vi "QI_correlation_X.vi"(6 "拟合半径":i32=5, 11 "QI 传递变量":T1) -> (3 "最相关位置":dbl)   [LabVIEW 2017]
doc: "本VI是QI算法中的核心部分之一，用途在于将x轴上的radial profile 连起来，并和自己的反向做相关性计算，得到相关性曲线后，在最大相关位置附近做二次方程拟合，计算出顶点的坐标，再结合图心坐标做出修正，从而得到小球的xy值，并在下一次测量前修正ROI的位置。\n本VI有一些需要注释的地方，便于后面的调试者理解。\n1、在拼接x轴左边和右边的radial profile前，在中间加了一个0值，这是因为算强度分布的时候没有计算0点的值，如果不补，可能后面会造成坐标的错位，0点的值是不重要的，反正哪个方向的0点值都应该一致，就取默认值即可。\n2、由于相关值算出来比较大，为了简化计算量，对负相关进行了有偏修正，无偏修正的结果似乎很奇怪，不能采用。\n3、拟合半径的设计是基于负相关曲线不是一个单纯的双曲线，由于衍射环有多个亮环，相关曲线也是波浪形，只有对最相关位置的附近做二次拟合才是合适的，对全局拟合的话，其他不是二次分布的点会降低拟合的可信度。拟合半径的默认值是5，应该可以应付大多数情况。\n4、为了达到超越像素的精度，我们直接用拟合的系数计算得到了顶点的x坐标，从而得出最相关位置。\n5、程序框图禁用的部分是调试时使用的显示图之类的，结束调试后应该重新禁用，否则这部分会吃内存并且影响速度。"
uses:
  <vilib>/Analysis/2dsp.llb/1D Cross Correlation (DBL).vi
  <vilib>/Analysis/NI_AALPro.lvlib
panel:
  out "相关曲线":cluster{dbl[], "Best Polynomial Fit":dbl[]}[](graph)
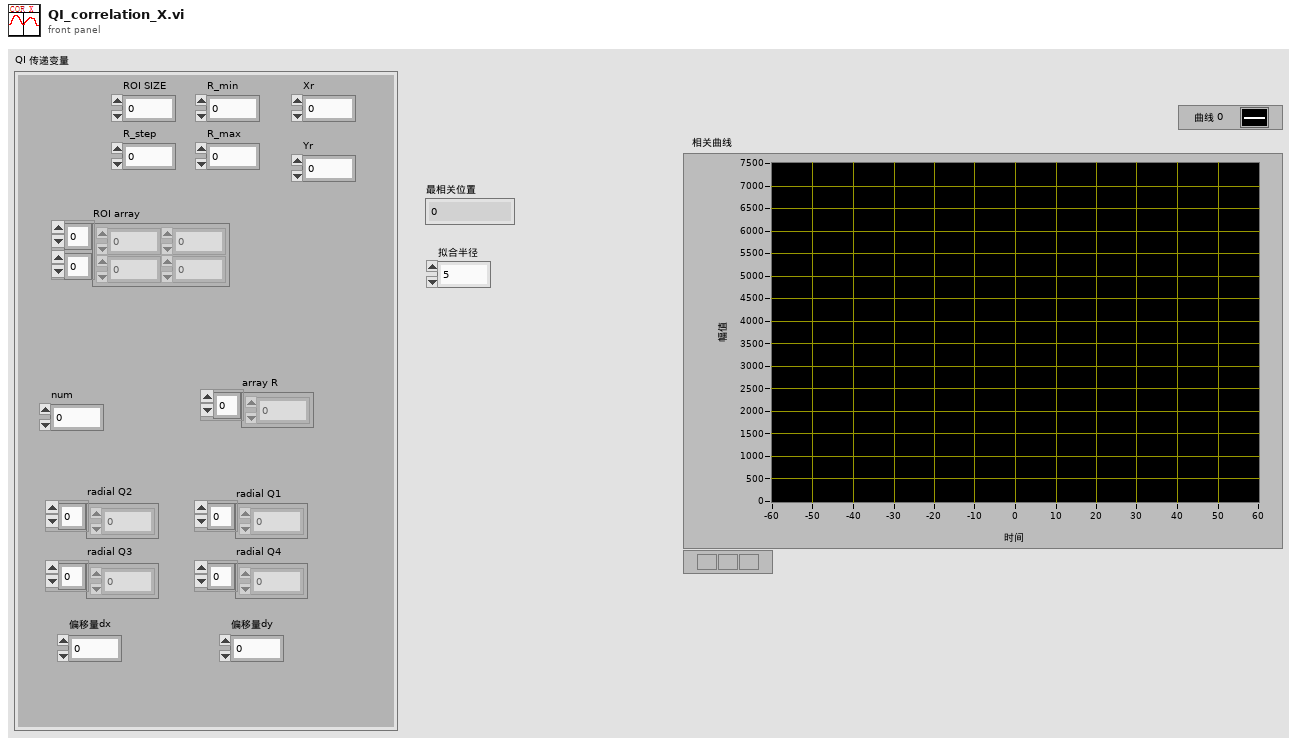
[diagram p1: front panel]
types:
  T1 = typedef "QI 传递变量.ctl" = cluster{"ROI SIZE":i32, "R_step":dbl, "R_min":dbl, "R_max":dbl, "num":dbl, "array R":dbl[], "radial Q1":dbl[], "radial Q2":dbl[], "radial Q3":dbl[], "radial Q4":dbl[], "偏移量dx":dbl, "偏移量dy":dbl, "ROI array":sgl[][], "Xr":dbl, "Yr":dbl}
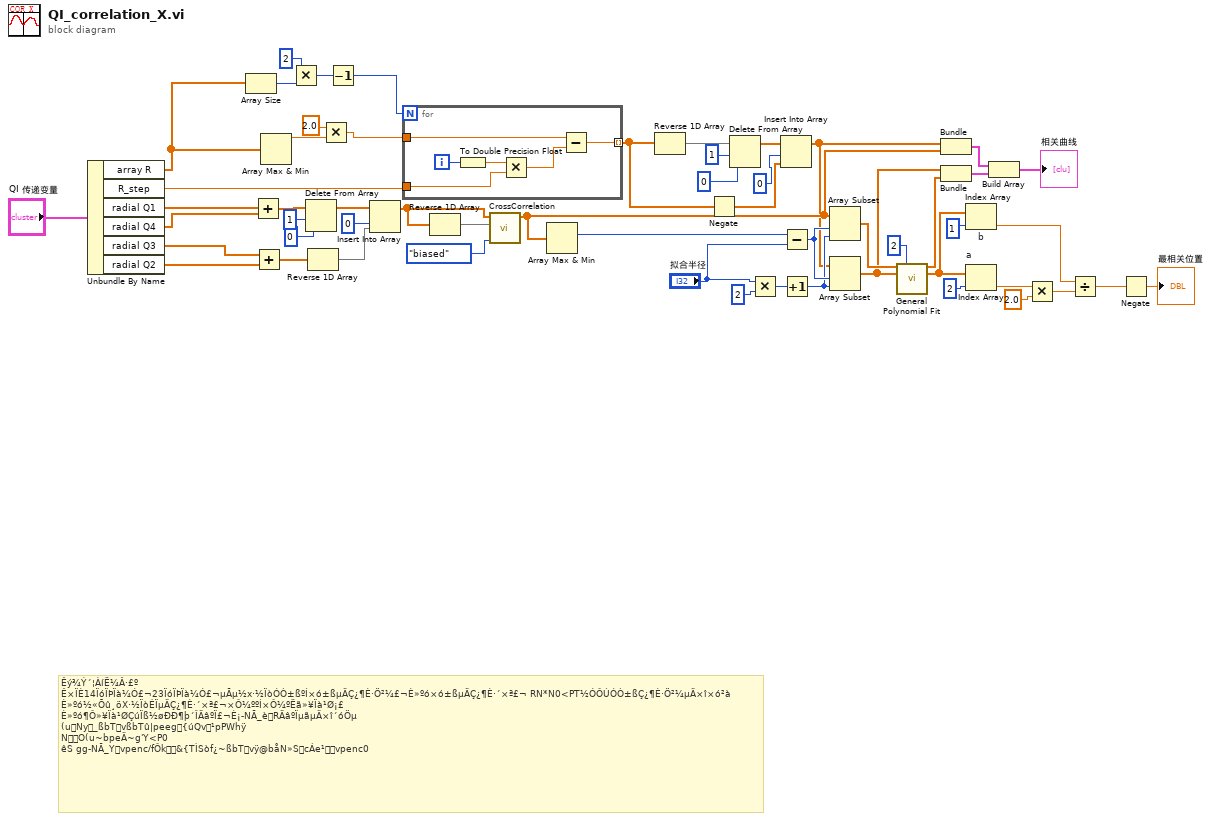
[diagram p0: block diagram]
diagram:
  # "Êý¾Ý´¦ÀíË¼Â·£º\nÊ×ÏÈ14ÏóÏÞÏà¼Ó£¬23ÏóÏÞÏà¼Ó£¬µÃµ½x·½ÏòÓÒ±ßºÍ×ó±ßµÄÇ¿¶È·Ö²¼£¬È»ºó×ó±ßµÄÇ¿¶È·´×ª£¬ RN*N0<PT½ÓÔÚÓÒ±ßÇ¿¶È·Ö²¼µÄ×î×ó²à\nÈ»ºó½«Õû¸öX·½ÏòÉÏµÄÇ¿¶È·´×ª£¬×Ô¼ººÍ×Ô¼ºËã»¥Ïà¹Ø¡£\nÈ»ºó¶Ô»¥Ïà¹ØÇúÏß½øÐÐ¶þ´ÎÄâºÏ£¬È¡-NÃ_èRÄâºÏµãµÄ×î´óÖµ\n(uNy_ßbTvßbTû|peeg{úQv¹pPWhÿ\nNO(u~bpeÄ~g'Y<P0\nêS\tgg-NÃ_Yvpenc/fÔk&{TÌSòf¿~ßbTvÿ@båN»ScÁe¹vpenc0"
  n1 = Unbundle By Name("QI 传递变量") -> ("array R"=w12:dbl[], "R_step"=w11:dbl, "radial Q1"=w52:dbl[], "radial Q4"=w7:dbl[], "radial Q3"=w5:dbl[], "radial Q2"=w6:dbl[])
  n2 = Array Size(array=w12) -> (size(s)=w15:i32)
  n3 = Add(x=w52, y=w7) -> (x+y=w10:dbl[])
  n4 = Add(x=w5, y=w6) -> (x+y=w53:dbl[])
  n5 = Array Max & Min(array=w12) -> (max value=w27:dbl)  [unwired: 3 out]
  n6 = Multiply(x=2, y=w15) -> (x*y=w13:i32)
  n7 = Delete From Array(array=w10, length=1 ("长度"), index=0 ("索引")) -> (array with subset deleted=w4:dbl[])  [unwired: 1 out]
  n8 = Reverse 1D Array(array=w53) -> (reversed array=w39:dbl[])
  n9 = Multiply(x=2.0, y=w27) -> (x*y=w3:dbl)
  n10 = Decrement(x=w13) -> (x-1=w2:i32)
  n11 = Insert Into Array(array=w4, index=0 ("索引"), new element=w39) -> (w35:dbl[])
  n12 = for "For循环" {
    N: w2 -> [_]
    tunnel: [w60] -> w22 mode=indexing
    tunnel: w3 -> [w56]
    tunnel: w11 -> [w58]
    i -> [w61]
    n13 = To Double Precision Float(number=w61) -> (double precision float=w57:dbl)
    n14 = Multiply(x=w57, y=w58) -> (x*y=w59:dbl)
    n15 = Subtract(x=w56, y=w59) -> (x-y=w60:dbl)
  }
  n16 = Reverse 1D Array(array=w35) -> (reversed array=w36:dbl[])
  n17 = call-poly <vilib>:"CrossCorrelation.vi"("normalization"=enum32{"none", "unbiased", "biased"}."biased", "Y"=w36, "X"=w35) -> ("Rxy"=w37:dbl[])  [unwired: 7 in, 1 out]
  n18 = Array Max & Min(array=w37) -> (max index (indices)=w34:i32)  [unwired: 3 out]
  n19 = Reverse 1D Array(array=w22) -> (reversed array=w18:dbl[])
  n20 = Negate(x=w22) -> (-x=w17:dbl[])
  n21 = Delete From Array(array=w18, length=1 ("索引"), index=0 ("索引")) -> (array with subset deleted=w21:dbl[])  [unwired: 1 out]
  n22 = Multiply(x="拟合半径", y=2 ("x")) -> (x*y=w32:i32)
  n23 = Insert Into Array(array=w21, index=0 ("索引"), new element=w17) -> (w16:dbl[])
  n24 = Subtract(x=w34, y="拟合半径") -> (x-y=w25:i32)
  n25 = Increment(x=w32) -> (x+1=w24:i32)
  n26 = Array Subset(array=w37, index=w25, length=w24) -> (w40:dbl[])
  n27 = Array Subset(array=w16, index=w25, length=w24) -> (w23:dbl[])
  n28 = call <vilib>:"General Polynomial Fit.vi"("Y"=w40, "polynomial order"=2, "X"=w23) -> ("Best Polynomial Fit"=w50:dbl[], "Polynomial Coefficients"=w48:dbl[])  [unwired: 9 in, 2 out]
  n29 = Bundle(w16, "Rxy"=w37) -> (w30:cluster{dbl[], "Rxy":dbl[]})  [unwired: 1 in]
  n30 = Bundle(w23, "Best Polynomial Fit"=w50) -> (w29:cluster{dbl[], "Best Polynomial Fit":dbl[]})  [unwired: 1 in]
  n31 = Index Array "b"(array=w48, index=1 ("索引")) -> (element=w44:dbl)
  n32 = Index Array "a"(array=w48, index=2 ("索引")) -> (element=w46:dbl)
  n33 = Build Array(w30, w29) -> (→"相关曲线":cluster{dbl[], "Best Polynomial Fit":dbl[]}[])
  n34 = Multiply(x=w46, y=2.0) -> (x*y=w43:dbl)
  n35 = Divide(x=w44, y=w43) -> (x/y=w42:dbl)
  n36 = Negate(x=w42) -> (-x=→"最相关位置":dbl)
